vi "CPU_MEM_CIA 2.vi"(7 "oper":enum16{"init", "read", "write"}(ring), 10 "value in":u8 format="%02x", 11 "address":u16 format="%04x") -> (2 "value out":u8 format="%02x")   [LabVIEW 2018]
panel:
  in  "init size":u16=15 format="%.0x"
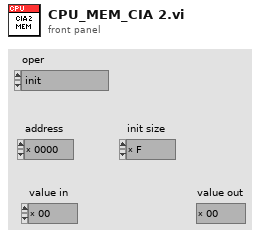
[diagram p1: front panel]
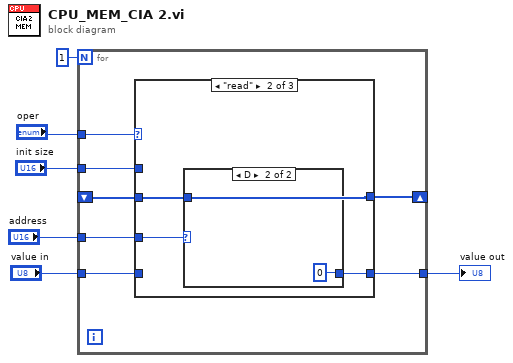
[diagram p0: block diagram]
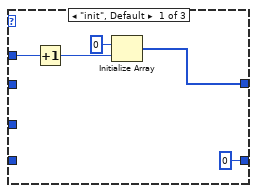
[diagram p2: hidden frame]
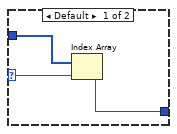
[diagram p3: hidden frame]
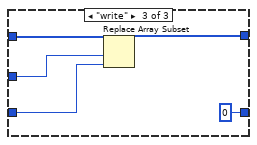
[diagram p4: hidden frame]
diagram:
  n1 = for {
    N: 1 -> [_]
    shift-right: [w11] -> _
    shift-left: _ -> [w10]
    tunnel: "oper" -> [w13]
    tunnel: "init size" -> [w12]
    tunnel: [w9] -> w3
    tunnel: "address" -> [w8]
    tunnel: "value in" -> [w7]
    n2 = case shown="\"read\"" w13 {
      tunnel: w12 -> [w18 _ _]
      tunnel: [w16 w21 w27] -> w11
      tunnel: w10 -> [_ w21 w30]
      tunnel: [u8 0 ("element") w20 u8 0 ("element")] -> w9
      tunnel: w8 -> [_ w19 w29]
      tunnel: w7 -> [_ _ w28]
      frame "init", Default {
        n3 = Increment(x=w18) -> (x+1=w14:u16)
        n4 = Initialize Array(u8 0 ("element"), w14) -> (w16:u8[])
      }
      frame "read" {
        n5 = case shown="D" w19 {
          selector: w19 -> [w22 _]
          tunnel: w21 -> [w24 _]
          tunnel: [w23 u8 0 ("element")] -> w20
          frame Default {
            n6 = Index Array(array=w24, index=w22) -> (element=w23:u8)
          }
          frame 13 {
          }
        }
      }
      frame "write" {
        n7 = Replace Array Subset(array=w30, new element=w28, index=w29) -> (w27:u8[])
      }
    }
  }
  "value out" <- w3
